vi "SA5G_EVM_Optimize.vi"(7 "Wait(ms)":u32=2000, 8 "error in":errorcluster, 11 "VISA in":refnum<visa-resource-name>) -> (0 "error out":errorcluster, 3 "VISA out":refnum<visa-resource-name>)   [LabVIEW 2020, in "Keysight.lvlib"]
uses:
  Keysight.lvlib
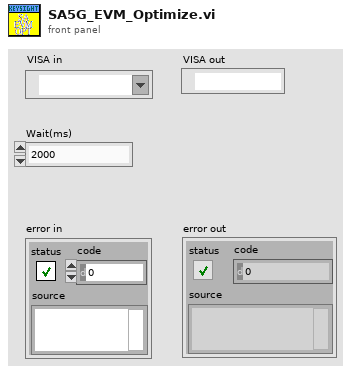
[diagram p1: front panel]
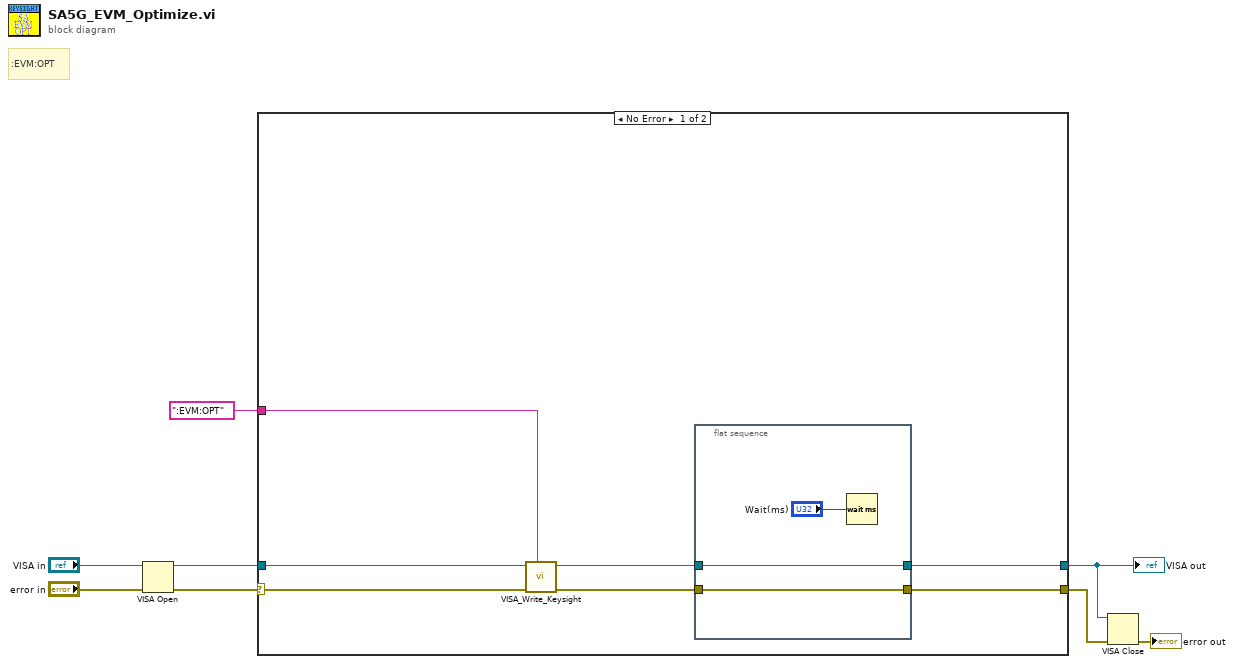
[diagram p0: block diagram]
diagram:
  # ":EVM:OPT"
  n1 = VISA Open(error in (no error)="error in", VISA resource name="VISA in") -> (VISA resource name=w3:refnum<visa-resource-name>, error out=w5:errorcluster)  [unwired: 3 in]
  n2 = case shown="No Error" w5 {
    selector: w5 -> [w14 w20]
    tunnel: [w11 w20] -> w8
    tunnel: [w9 w19] -> w1
    tunnel: ":EVM:OPT" ("write buffer") -> [w15 _]
    tunnel: w3 -> [w13 w19]
    frame No Error {
      n3 = call "VISA_Write_Keysight.vi"("VISA CMD"=w15, "error in"=w14, "VISA in"=w13) -> ("error out"=w12:errorcluster, "VISA out"=w10:refnum<visa-resource-name>)  [unwired: 7 in]
      n4 = flat-sequence {
        tunnel: w12 -> [w18]
        tunnel: [w18] -> w11
        tunnel: w10 -> [w17]
        tunnel: [w17] -> w9
        frame #0 {
          n5 = Wait (ms)(milliseconds to wait="Wait(ms)") -> ()  [unwired: 1 out]
        }
      }
    }
    frame Error {
    }
  }
  "VISA out" <- w1
  n6 = VISA Close(VISA resource name=w1, error in (no error)=w8) -> (error out=→"error out":errorcluster)
